vi "calcutateFuturePointToTable.vi"(4 "OffensivePlay":T1, 6 "BallRef":refnum<class "Ball.lvclass">, 7 "AttackingOurselves?":bool=TRUE, 8 "error in (no error)":errorcluster, 9 "Robot that\nmake the pass":refnum<class "Robot.lvclass">, 10 "Robot that will\nreceive the pass":refnum<class "Robot.lvclass">, 11 "KickToPassReceiverTactic in":refnum<class "KickToPassReceiverTactic.lvclass">) -> (0 "error out":errorcluster, 2 "Array to Receiver trajectory":dbl[](array[numeric]), 3 "KickToPassReceiverTactic out":refnum<class "KickToPassReceiverTactic.lvclass">)   [LabVIEW 2023, in "KickToPassReceiverTactic.lvclass"]
uses:
  KickToPassReceiverTactic.lvclass
  Ball_class/Ball.lvclass
  Robot_class/Robot.lvclass
  Team_class/OffensivePlay.ctl
  Robot_class/Robot.lvclass/Robot.ctl
  Object_class/Object.lvclass/Object.ctl
  Utilities_class/Utilities.lvclass
  <vilib>/Analysis/coordinate.llb/2D Cartesian Coordinate Rotation (Scalar).vi
  Object_class/Read x.vi
  Object_class/Read y.vi
  Robot_class/Read role.vi
  <vilib>/Analysis/NI_AALPro.lvlib
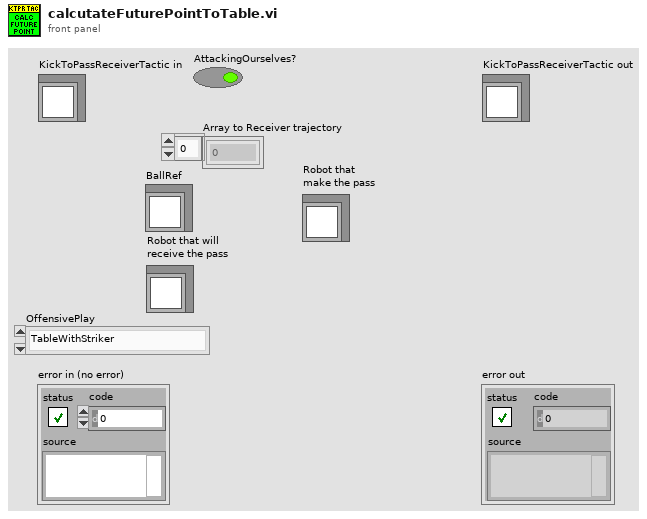
[diagram p1: front panel]
types:
  T1 = typedef "OffensivePlay.ctl" = enum16{"TableWithStriker", "TableWith2ndStrikerPlay", "PrepareDoublePass", "PrepareRollToPass", "SimplePass", "PreparePass", "PassToStriker", "BallOutOfField", "PassTo2ndStriker", "StopOffensive", "Prepare Penalty Enemy", "EnemyPossessionAtEnemyField", "EnemyPossesionAtOurField", "TestPlay", "PreparePenaltyAlly", "KickPenaltyAlly", "PrepareKickoffAlly", "PrepareKickoffEnemy", "IndirectEnemy", "DirectEnemy", "NormalGame", "DirectKick", "Pass", "Halt", "Timeout", "PassPlay", "PenaltyEnemy"}
  T2 = typedef "roles.ctl" = enum16{"BallChallengerAttackerVSS", "NormalAttackerVSS", "AttackerAimGoalVSS", "DefenderAreaVSS", "KeeperVSS", "Tabler", "TableFinalizer", "PrepareRollToPassRoller", "PrepareRollToPassReceiver", "SimplePassRoll", "SimplePassRollReceiver", "PenaltyDefense", "PreparePassReceiver 2", "PreparePassReceiver 1", "PassObserver", "Timeout", "Goto", "ZigZag", "None", "BallOutOfField", "DefenderArea", "Duelist", "AttackerStop", "FollowAttacker", "KeeperRole", "KickPenalty", "AttackerAimGoal", "AttackerBlock", "Marker", "Halt", "Shoot", "PassKicker", "PassReceiver", "TestRole", "PenaltyAttacker"}
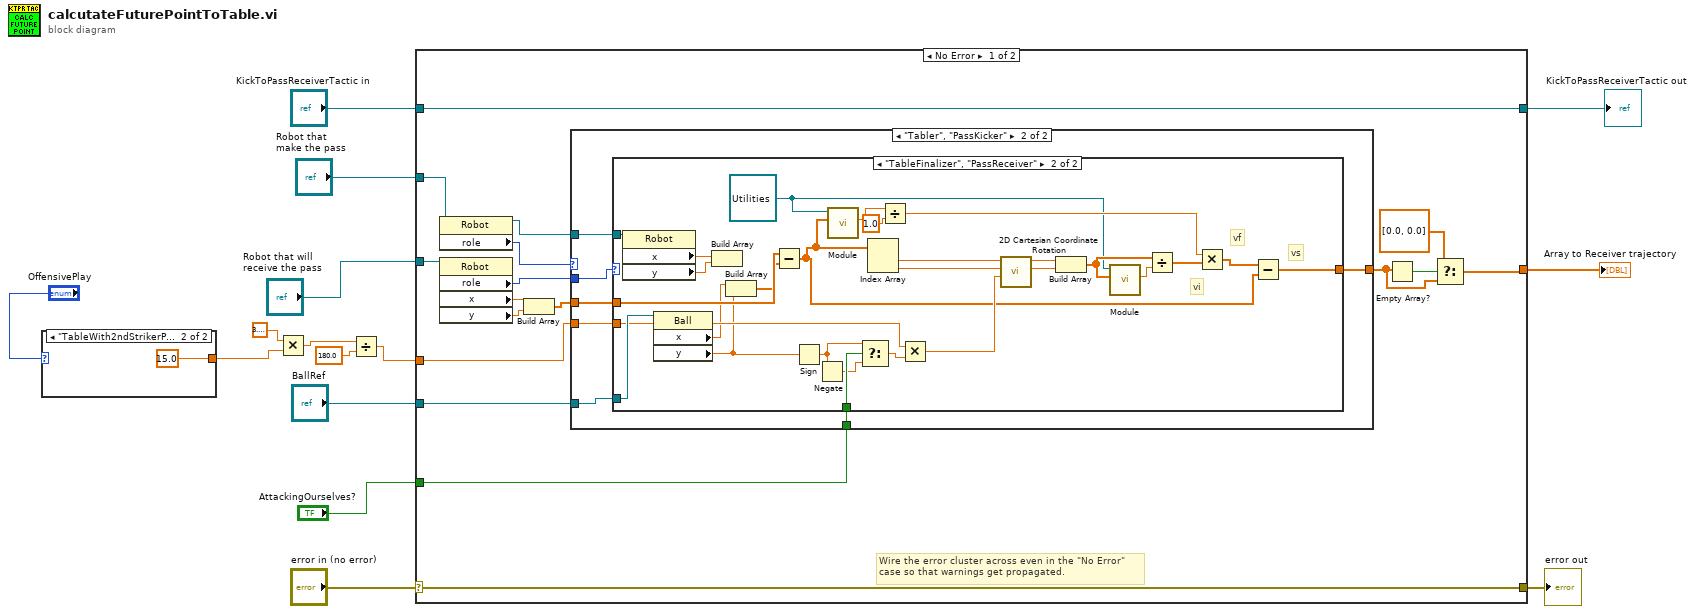
[diagram p0: block diagram]
diagram:
  n1 = case shown="\"TableWith2ndStrikerPlay\"" "OffensivePlay" {
    tunnel: [_ 15.0] -> w5
    frame "TableWithStriker", Default {
    }
    frame "TableWith2ndStrikerPlay" {
    }
  }
  n2 = Multiply(x=3.141592653589793, y=w5) -> (x*y=w4:dbl)
  n3 = Divide(x=w4, y=180.0) -> (x/y=w2:dbl)
  n4 = case shown="No Error" "error in (no error)" {
    selector: "error in (no error)" -> [w32 w70]
    tunnel: [w32 w70] -> w14
    tunnel: [w33 w69] -> w12
    tunnel: "KickToPassReceiverTactic in" -> [w33 w69]
    tunnel: "BallRef" -> [w31 _]
    tunnel: w2 -> [w30 _]
    tunnel: "AttackingOurselves?" -> [w29 _]
    tunnel: [w25 _] -> w9
    tunnel: "Robot that\nmake the pass" -> [w24 _]
    tunnel: "Robot that will\nreceive the pass" -> [w21 _]
    frame No Error {
      # "Wire the error cluster across even in the \"No Error\"\ncase so that warnings get propagated."
      n5 = property class="Robot"(reference=w24) -> (reference out=w22:refnum<class "Robot.lvclass">, "role"=w23:T2)  [unwired: 1 in, 1 out]
      n6 = property class="Robot"(reference=w21) -> ("role"=w20:T2, "x"=w18:dbl, "y"=w17:dbl)  [unwired: 1 in, 2 out]
      n7 = Build Array(w18, w17) -> (w19:dbl[])
      n8 = case shown="\"Tabler\", \"PassKicker\"" w23 {
        tunnel: w20 -> [_ w40]
        tunnel: w19 -> [_ w39]
        tunnel: w31 -> [_ w38]
        tunnel: w30 -> [_ w37]
        tunnel: w29 -> [_ w36]
        tunnel: [_ w35] -> w27
        tunnel: w22 -> [_ w34]
        frame Default {
        }
        frame "Tabler", "PassKicker" {
          n9 = case shown="\"TableFinalizer\", \"PassReceiver\"" w40 {
            tunnel: w39 -> [_ w54]
            tunnel: w38 -> [_ w66]
            tunnel: w37 -> [_ w65]
            tunnel: w36 -> [_ w64]
            tunnel: [_ w53] -> w35
            tunnel: w34 -> [_ w57]
            frame Default {
            }
            frame "TableFinalizer", "PassReceiver" {
              w44 = refnum<class "Utilities.lvclass"> refnum ("Utilities in")
              # "vi"
              # "vs"
              # "vf"
              n10 = property class="Robot"(reference=w57) -> ("x"=w56:dbl, "y"=w55:dbl)  [unwired: 1 in, 2 out]
              n11 = property class="Ball"(reference=w66) -> ("x"=w43:dbl, "y"=w42:dbl)  [unwired: 1 in, 2 out]
              n12 = Build Array(w56, w55) -> ()  [unwired: 1 out]
              n13 = Build Array(w43, w42) -> (w41:dbl[])
              n14 = Subtract(x=w54, y=w41) -> (x-y=w48:dbl[])
              n15 = Sign(1:w42) -> (0:w62:dbl)
              n16 = Negate(x=w62) -> (-x=w63:dbl)
              n17 = call-dynamic "Module.vi"("2D vector"=w48, "Utilities in"=w44) -> ("Modulo"=w47:dbl)  [unwired: 7 in, 2 out]
              n18 = Select(t=w62, s=w64, f=w63) -> (s? t:f=w61:dbl)
              n19 = Index Array(array=w48) -> (element #1=w68:dbl, element #2=w67:dbl)  [unwired: 2 in]
              n20 = Divide(x=w47, y=1.0) -> (x/y=w45:dbl)
              n21 = Multiply(x=w65, y=w61) -> (x*y=w60:dbl)
              n22 = call-poly <vilib>:"2D Cartesian Coordinate Rotation.vi"("theta"=w60, "y"=w67, "x"=w68) -> ("y out"=w58:dbl, "x out"=w59:dbl)  [unwired: 6 in, 1 out]
              n23 = Build Array(w59, w58) -> (w52:dbl[])
              n24 = call-dynamic "Module.vi"("2D vector"=w52, "Utilities in"=w44) -> ("Modulo"=w51:dbl)  [unwired: 7 in, 2 out]
              n25 = Divide(x=w52, y=w51) -> (x/y=w50:dbl[])
              n26 = Multiply(x=w45, y=w50) -> (x*y=w49:dbl[])
              n27 = Subtract(x=w49, y=w48) -> (x-y=w53:dbl[])
            }
          }
        }
      }
      n28 = Empty Array?(array=w27) -> (empty?=w28:bool)
      n29 = Select(t=dbl[] [0.0, 0.0], s=w28, f=w27) -> (s? t:f=w25:dbl[])
    }
    frame Error {
    }
  }
  "error out" <- w14
  "KickToPassReceiverTactic out" <- w12
  "Array to Receiver trajectory" <- w9
